vi "SUBVI_rate.vi"(7 "Refresco(s)":dbl=5.0 caption="Elapsed Time (s)", 8 "Error In":errorcluster) -> (0 "Error Out":errorcluster, 3 "Nuevo?":bool, 5 "Remote?":bool)   [LabVIEW 2013]
doc: "Illustrates how to create and write a configuration settings file.\n\nInstructions:\nEnter values in the controls on the front panel then click on the Run Arrow.\nTo read the file, run Read Configuration Settings File.vi located in the file\\config.llb."
uses:
  datosGraficaRateNumeric.ctl
  datosGraficaRateString.ctl
  ANAIS_GLOBALES.vi
panel:
  out "rateString":T1
  out "ratenum":T2 {"FreqRun" format="%.1f"; "Frequency" format="%.1f"; "Time" format="%.1f"; "TotalBlocks" format="%.1f"; "Block" format="%.1f"}
  out "SUM=0?":bool
  out "Errores acum S":i32 caption="Elapsed Time (s)"
  out "Errores acum W":i32 caption="Elapsed Time (s)"
  out "Web":string caption="asd"
  out "Idx":i32 caption="Elapsed Time (s)"
  in  "stop":bool
  out "Date":string caption="asd"
  out "Time":string caption="asd"
  in  "Refresh":bool
  # "Monitor de frecuencia de sucesos"
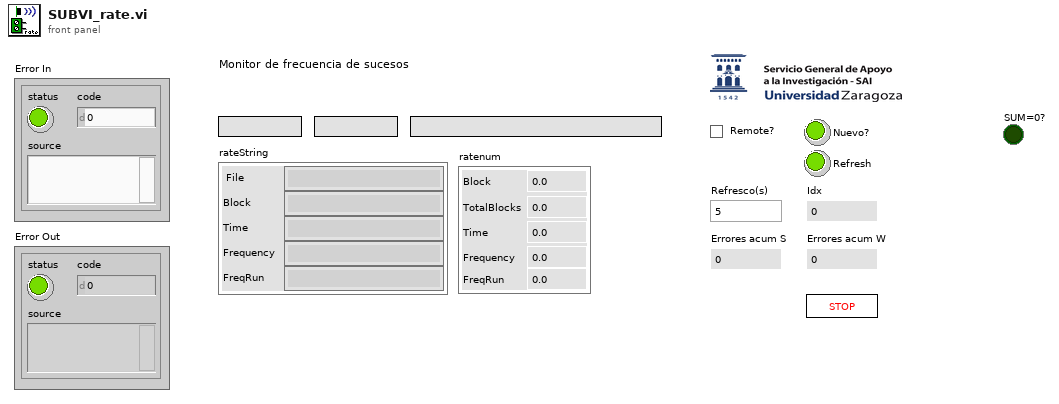
[diagram p1: front panel]
types:
  T1 = typedef "datosGraficaRateString.ctl" = cluster{" File":string, "Block":string, "Time":string, "Frequency":string, "FreqRun":string}
  T2 = typedef "datosGraficaRateNumeric.ctl" = cluster{"Block":dbl, "TotalBlocks":dbl, "Time":dbl, "Frequency":dbl, "FreqRun":dbl}
  T3 = typedef "puertosIP.ctl" = cluster{"IMonWeb":string, "IMon":bool, "VMonWeb":string, "VMon":bool, "ClimatWeb":string, "Climat":bool, "RadonWeb":string, "Radon":bool, "BeagleEWeb":string, "BeagleE":bool, "BeagleDWeb":string, "BeagleD":bool, "RateWeb":string, "Rate":bool, "CratesWeb":string, "Crates":bool, "StartStopWeb":string, "StartStop":bool, "MuonRatesWeb":string, "MuonRates":bool, "N2LIQWeb":string, "N2LIQ":bool}
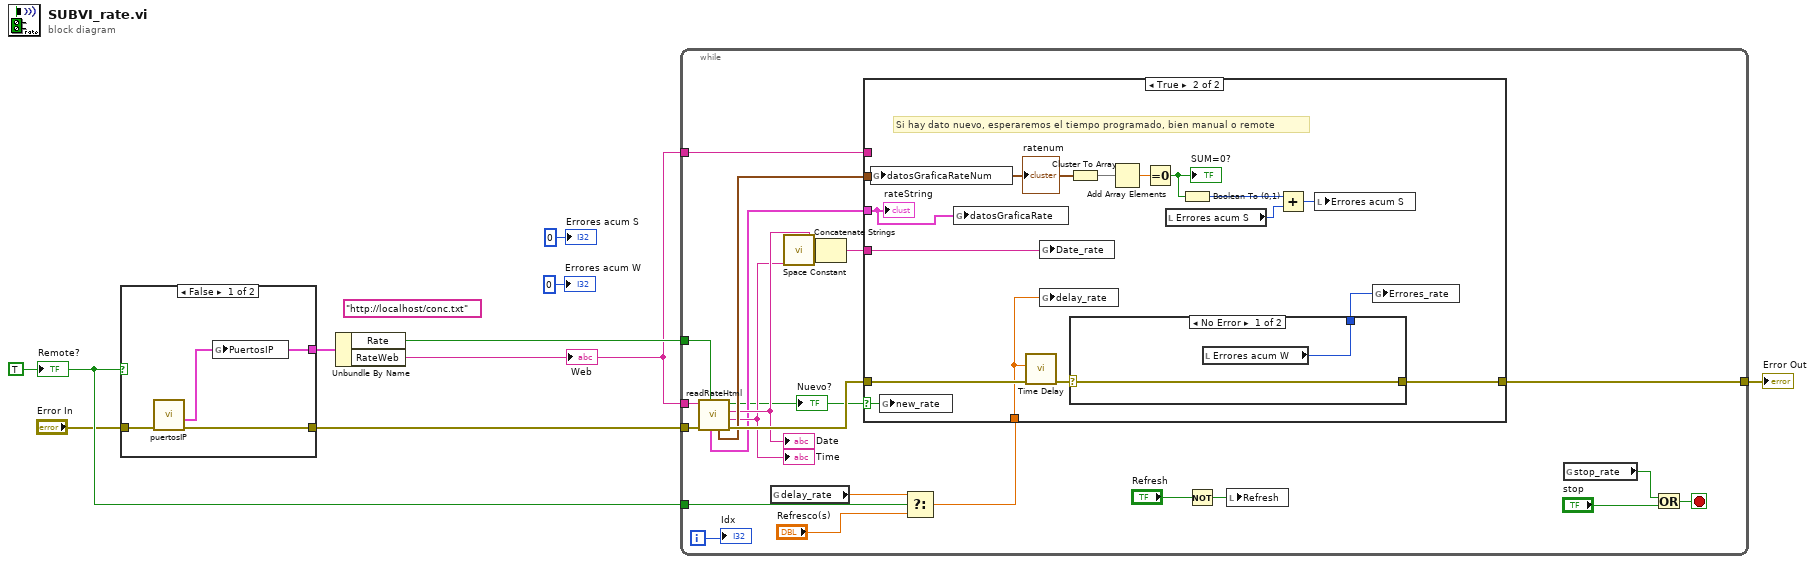
[diagram p0: block diagram]
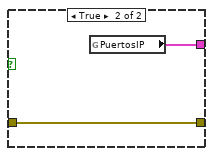
[diagram p2: hidden frame]
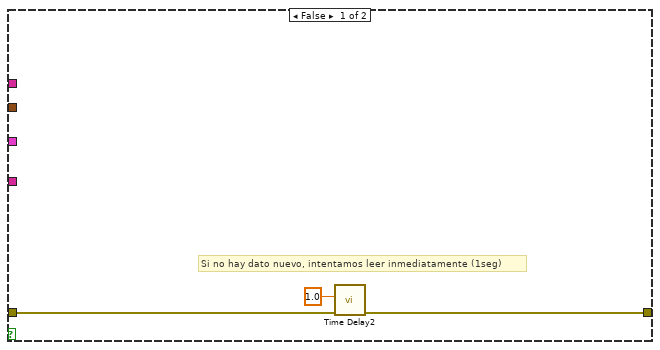
[diagram p3: hidden frame]
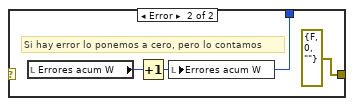
[diagram p4: hidden frame]
diagram:
  (unwired) "http://localhost/conc.txt" ("Web")
  w6 = TRUE ("Remote?")
  n1 = case shown="False" w6 {
    tunnel: [w12 w14] -> w8
    tunnel: "Error In" -> [w10 w13]
    tunnel: [w11 w13] -> w2
    frame False {
      n2 = call "puertosIP.vi"("error in (no error)"=w10) -> ("error out"=w11:errorcluster, "Cluster"=w12:T3)  [unwired: 8 in, 1 out]
      n3 = global write "ANAIS_GLOBALES.vi" "PuertosIP"(w12) -> ()
    }
    frame True {
      n4 = global read "ANAIS_GLOBALES.vi" "PuertosIP"() -> (w14:T3)
    }
  }
  n5 = Unbundle By Name(w8) -> ("Rate"=w4:bool, "RateWeb"=w1:string)
  "Web" <- w1
  n6 = while {
    tunnel: [w18] -> w9
    tunnel: w6 -> [w29]
    tunnel: w1 -> [w28]
    tunnel: w2 -> [w26]
    tunnel: w1 -> [w25]
    tunnel: w4 -> [w24]
    i -> [w17]
    stop <- w34 stop-if-true
    n7 = call "readRateHtml.vi"("Web(T)"=w24, "Error In"=w26, "url"=w28) -> ("Error Out"=w27:errorcluster, "Hora"=w20:string, "Fecha"=w21:string, "datoNuevo?"=w15:bool, "datosGraficaRateNum"=w23:T2, "datosGraficaRate"=w16:T1)  [unwired: 2 in, 1 out]
    "Date" <- w21
    "Time" <- w20
    "Nuevo?" <- w15
    n8 = global read "ANAIS_GLOBALES.vi" "delay_rate"() -> (w30:dbl)
    n9 = call <vilib>:"Space Constant.vi"() -> ("String"=w22:string)
    n10 = Concatenate Strings(w21, w22, w20) -> (w19:string)
    n11 = Select(t=w30, s=w29, f="Refresco(s)") -> (s? t:f=w31:dbl)
    n12 = case shown="True" w15 {
      selector: w15 -> [_ w41]
      tunnel: w31 -> [_ w44]
      tunnel: w27 -> [w39 w55]
      tunnel: [w38 w53] -> w18
      tunnel: w25 -> [_ _]
      tunnel: w23 -> [_ w50]
      tunnel: w19 -> [_ w43]
      tunnel: w16 -> [_ w42]
      frame False {
        # "Si no hay dato nuevo, intentamos leer inmediatamente (1seg)"
        n13 = call "Time Delay2"("error in (no error)"=w39, "Delay Time (s)"=1.0) -> ("error out"=w38:errorcluster)  [unwired: 9 in]
      }
      frame True {
        # "Si hay dato nuevo, esperaremos el tiempo programado, bien manual o remote"
        n14 = global write "ANAIS_GLOBALES.vi" "datosGraficaRateNum"(w50) -> ()
        n15 = global write "ANAIS_GLOBALES.vi" "new_rate"(w41) -> ()
        n16 = global write "ANAIS_GLOBALES.vi" "datosGraficaRate"(w42) -> ()
        n17 = call "Time Delay"("error in (no error)"=w55, "Delay Time (s)"=w44) -> ("error out"=w54:errorcluster)  [unwired: 9 in]
        n18 = global write "ANAIS_GLOBALES.vi" "Date_rate"(w43) -> ()
        n19 = global write "ANAIS_GLOBALES.vi" "delay_rate"(w44) -> ()
        n20 = Cluster To Array(cluster=w50) -> (array=w49:dbl[])
        n21 = case shown="No Error" w54 {
          selector: w54 -> [w56 _]
          tunnel: [w56 errorcluster {"status"=FALSE, "code"=0, "source"=""} ("error IO")] -> w53
          tunnel: [w57 w59] -> w45
          frame No Error {
            n22 = local read "Errores acum W"() -> (w57:i32)
          }
          frame Error {
            # "Si hay error lo ponemos a cero, pero lo contamos"
            n23 = local read "Errores acum W"() -> (w60:i32)
            n24 = Increment(x=w60) -> (x+1=w59:i32)
            n25 = local write "Errores acum W"(w59) -> ()
          }
        }
        n26 = Add Array Elements(numeric array=w49) -> (sum=w52:dbl)
        n27 = Equal To 0?(x=w52) -> (x = 0?=w47:bool)
        "SUM=0?" <- w47
        n28 = local read "Errores acum S"() -> (w51:i32)
        n29 = Boolean To (0,1)(Boolean=w47) -> (0, 1=w46:i16)
        n30 = Add(x=w46, y=w51) -> (x+y=w48:i32)
        n31 = local write "Errores acum S"(w48) -> ()
        n32 = global write "ANAIS_GLOBALES.vi" "Errores_rate"(w45) -> ()
        "ratenum" <- w50
        "rateString" <- w42
      }
    }
    n33 = Not(x="Refresh") -> (.not. x?=w35:bool)
    n34 = local write "Refresh"(w35) -> ()
    n35 = global read "ANAIS_GLOBALES.vi" "stop_rate"() -> (w33:bool)
    n36 = Or(x=w33, y="stop") -> (x .or. y?=w34:bool)
    "Idx" <- w17
  }
  "Error Out" <- w9
  "Remote?" <- w6
  "Errores acum W" <- 0 ("Errores acum.")
  "Errores acum S" <- 0 ("Errores acum")
